vi "Example Callback - Station Data Callback.vi"(4 "StationData":refnum<user-event>, 5 "Event Data":T1, 6 "Control Ref":refnum<k24>, 7 "Event Common Data":T2) -> ()   [LabVIEW 2013]
uses:
  C:/tf/play/labview/Tinkerforge.dll
  Tinkerforge.dll
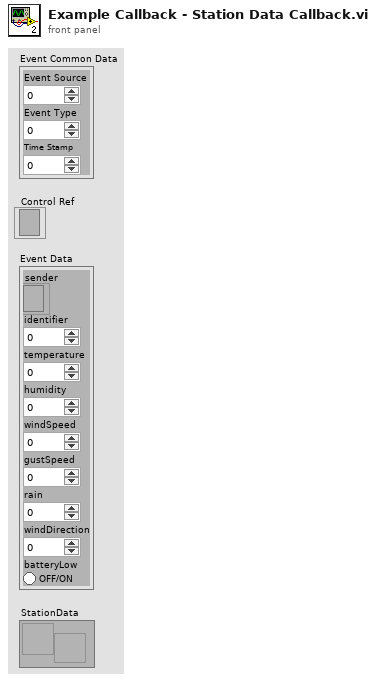
[diagram p1: front panel]
types:
  T1 = cluster{"sender":refnum<k24>, "identifier":u8, "temperature":i16, "humidity":u8, "windSpeed":i64, "gustSpeed":i64, "rain":i64, "windDirection":u8, "batteryLow":bool}
  T2 = cluster{"Event Source":i32, "Event Type":u32, "Time Stamp":u32}
  T3 = cluster{"identifier":u8, "temperature":i16, "humidity":u8, "windSpeed":i64, "gustSpeed":i64, "rain":i64, "windDirection":u8, "batteryLow":bool}
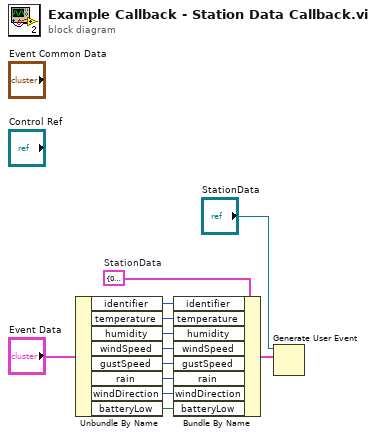
[diagram p0: block diagram]
diagram:
  w11 = T3 {"identifier"=0, "temperature"=0, "humidity"=0, "windSpeed"=0, "gustSpeed"=0, "rain"=0, "windDirection"=0, "batteryLow"=TRUE}  # StationData
  n1 = Unbundle By Name("Event Data") -> ("identifier"=w10:u8, "temperature"=w9:i16, "humidity"=w8:u8, "windSpeed"=w7:i64, "gustSpeed"=w6:i64, "rain"=w5:i64, "windDirection"=w4:u8, "batteryLow"=w3:bool)
  n2 = Bundle By Name(cluster=w11, "identifier"=w10, "temperature"=w9, "humidity"=w8, "windSpeed"=w7, "gustSpeed"=w6, "rain"=w5, "windDirection"=w4, "batteryLow"=w3) -> (w2:T3)
  n3 = Generate User Event(user event="StationData", event data cluster=w2) -> ()  [unwired: 2 in, 2 out]
